vi "Excel Example.vi"() -> ()   [LabVIEW 2017]
doc: "This example shows how to use the LabVIEW NPOI library to manipulate MS Excel Files."
uses:
  LabVIEW NPOI/MS-Excel/MS-Excel.lvclass
  Styles/Underline--ring.ctl
  Styles/Alignment--ring.ctl
  Styles/Font--cluster.ctl
  Styles/Style--cluster.ctl
  LabVIEW NPOI/Document/Read Table As String.vi
  9eaf8ef5-2da6-4511-8777-42b0d28acfa6.vi
  LabVIEW NPOI/Document/Append Table (double).vi
  <vilib>/Utility/sysdir.llb/System Directory Type.ctl
panel:
  in  "print":bool
  in  "HTML File Path":path
  in  "convertToHtml":bool
  out "Read Table Time":u32
  out "Add Table Time":u32
  in  "addImageBttn":bool
  in  "setActiveSheetBttn":bool
  out "Table Control":string[][](table)
  in  "readTableBttn":bool
  in  "Style":u16(ring)
  out "Current Sheet:Next Empty Cell":cluster{"Row":i32, "Column":i32}
  in  "#Columns":i32=100
  in  "#Rows":i32=2
  in  "tableType":enum32{"Strings", "Doubles"}(radio)
  in  "addTableBttn":bool
  in  "Set as active (T)":bool
  in  "addWorksheetBttn":bool
  out "Current Sheet:Name":string
  out "Workbook:Sheet List":string[](array[string])
  out "FilePath":path
  in  "openWorkbookBttn":bool
  in  "baseWorkbookPath":path caption="Folder Path"
  in  "saveAsWorkbookBttn":bool
  in  "saveWorkbookBttn":bool
  in  "removeSheetBttn":bool
  in  "workbookName":string="Book1.xlsx" caption="Name"
  in  "newWorksheetName":string caption="Sheet Name"
  in  "createWorkbookBttn":bool
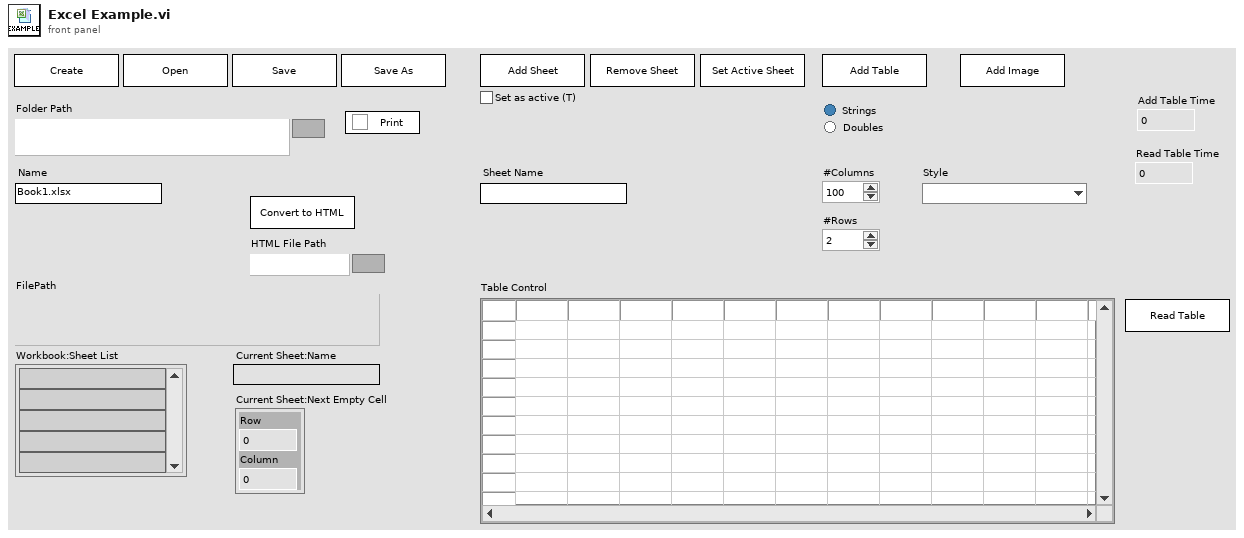
[diagram p1: front panel]
types:
  T1 = typedef "System Directory Type.ctl" = i32
  T2 = cluster{"workbookObject":refnum<class "MS-Excel.lvclass">, "workbookPath":path, "workbookName":string, "worksheetName":string, "styleName":string, "ctlRefs":refnum<vi>[]}
  T3 = typedef "Styles.lvlib/Style--cluster.ctl" = cluster{"Name":string, "Font":T4}
  T4 = typedef "Styles.lvlib/Font--cluster.ctl" = cluster{"Name":string, "Size":i32, "Bold":bool, "Italic":bool, "Underline":T5, "Strike":bool, "Color":u32, "Alignment":T6}
  T5 = typedef "Styles.lvlib/Underline--ring.ctl" = i32
  T6 = typedef "Styles.lvlib/Alignment--ring.ctl" = i32
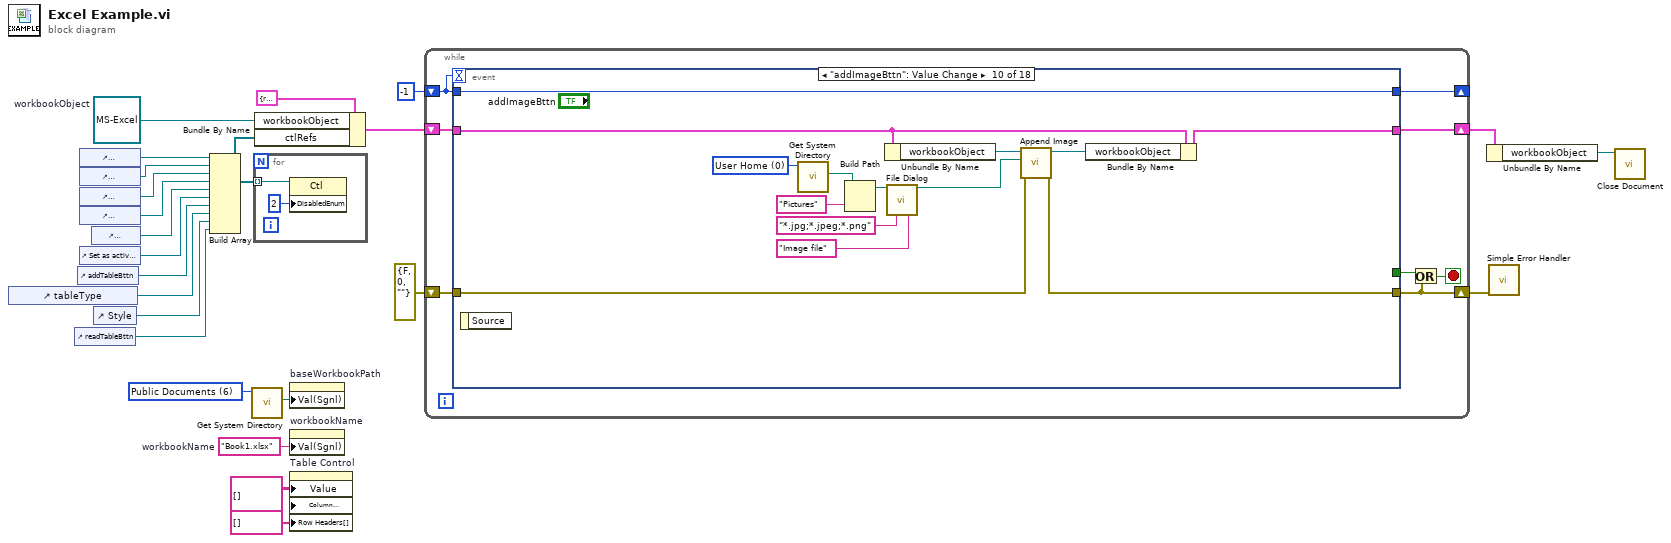
[diagram p0: block diagram]
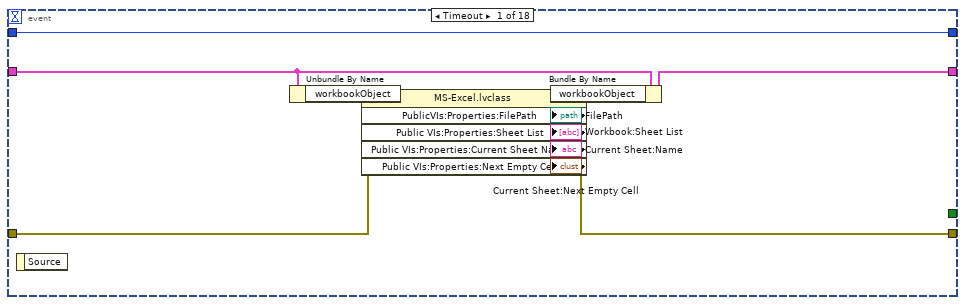
[diagram p2: hidden frame]
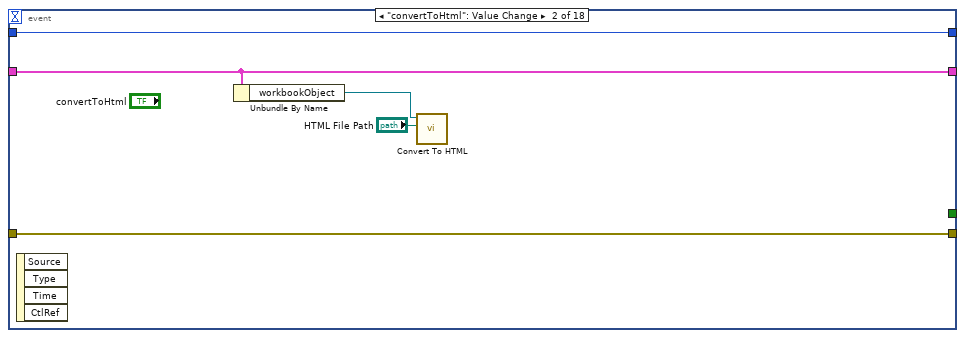
[diagram p3: hidden frame]
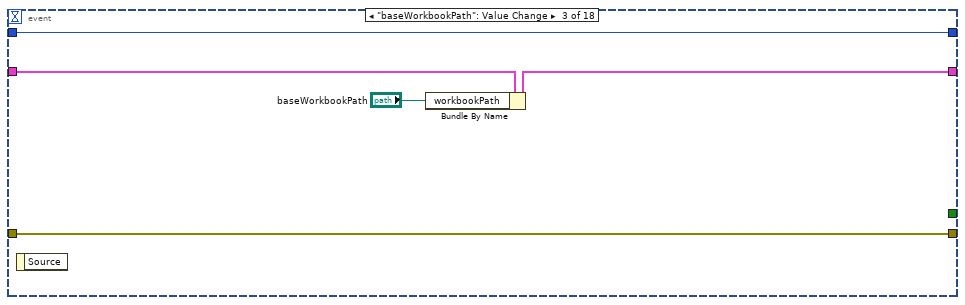
[diagram p4: hidden frame]
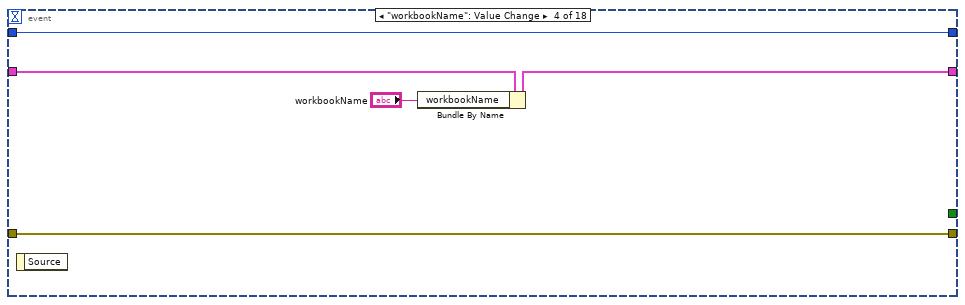
[diagram p5: hidden frame]
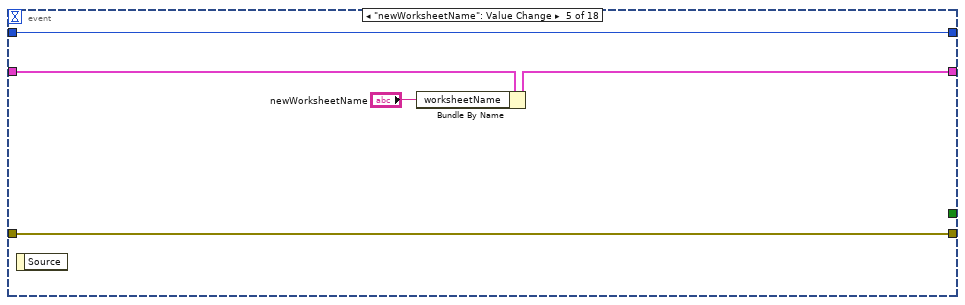
[diagram p6: hidden frame]
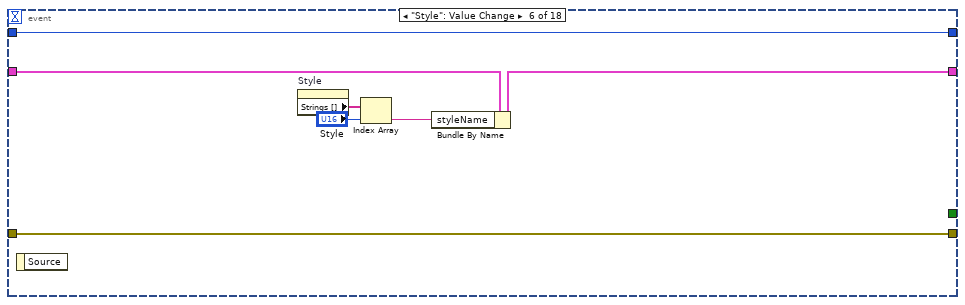
[diagram p7: hidden frame]
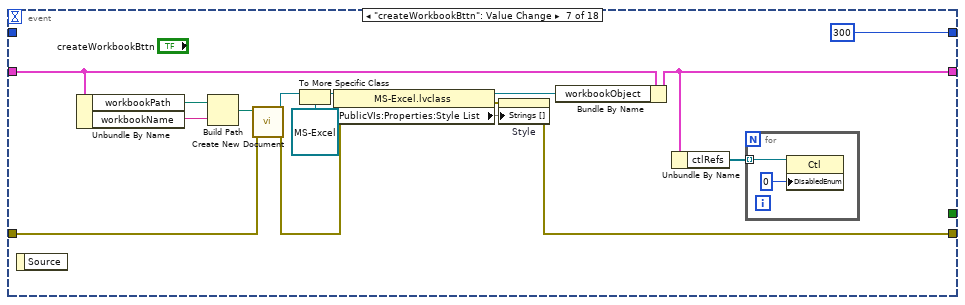
[diagram p8: hidden frame]
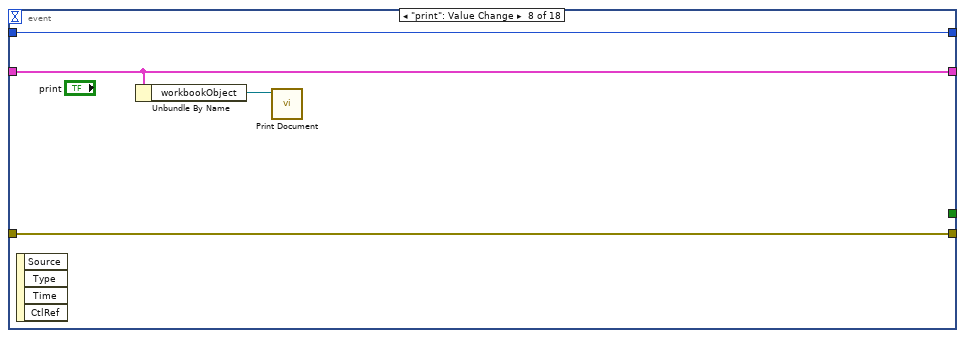
[diagram p9: hidden frame]
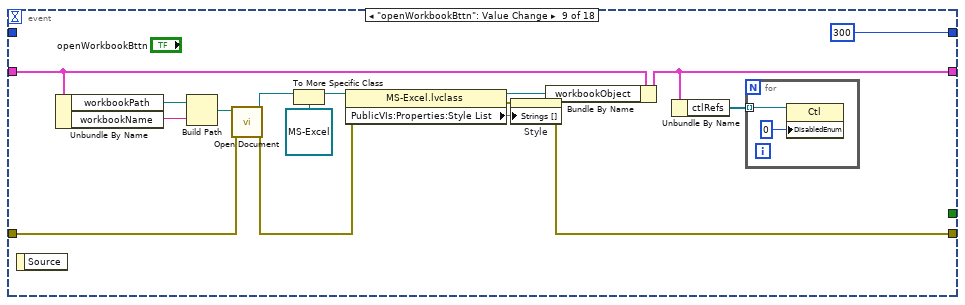
[diagram p10: hidden frame]
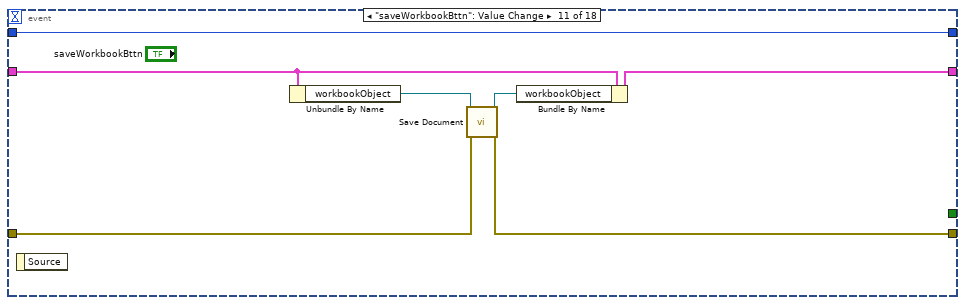
[diagram p11: hidden frame]
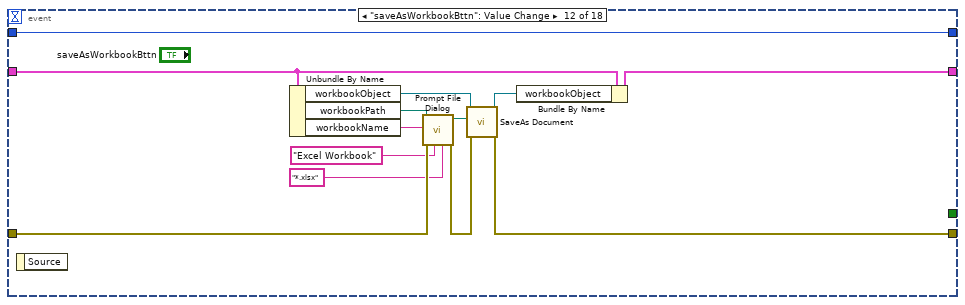
[diagram p12: hidden frame]
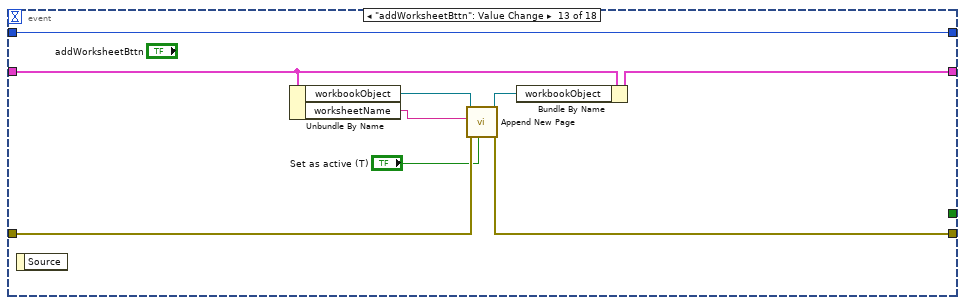
[diagram p13: hidden frame]
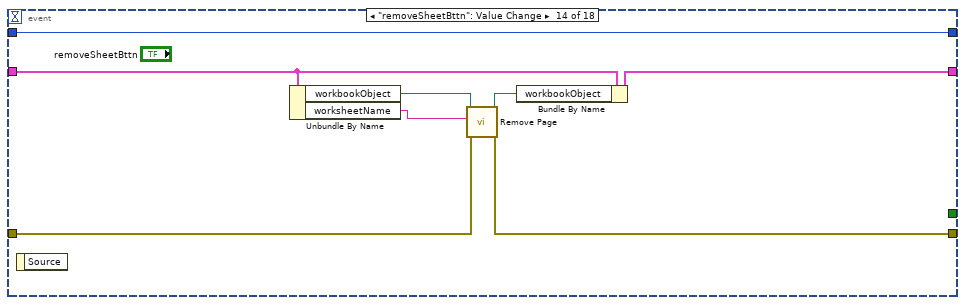
[diagram p14: hidden frame]
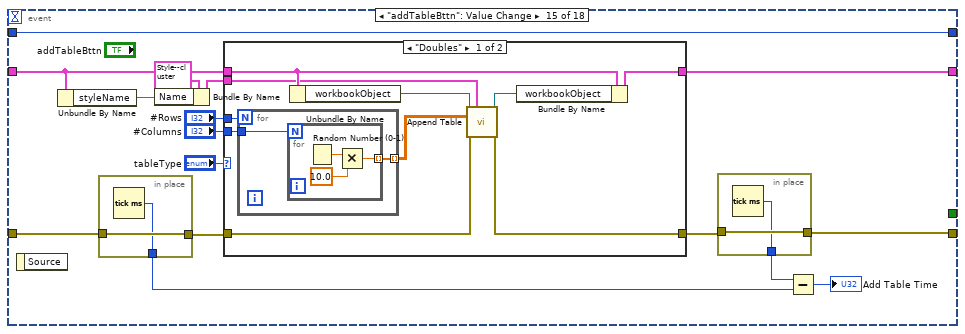
[diagram p15: hidden frame]
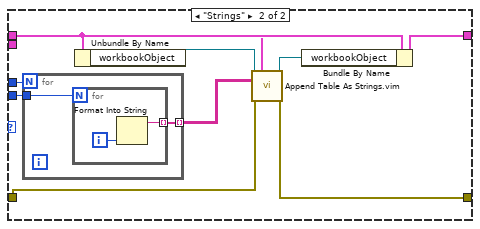
[diagram p16: hidden frame]
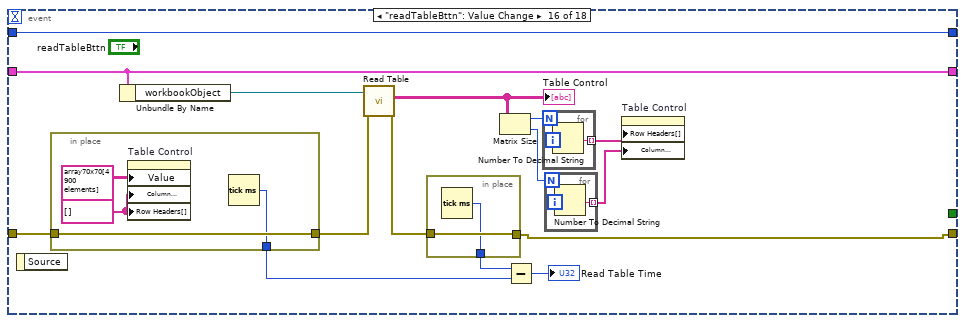
[diagram p17: hidden frame]
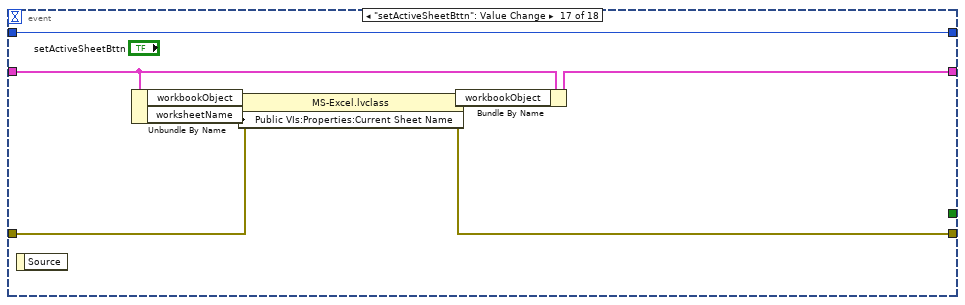
[diagram p18: hidden frame]
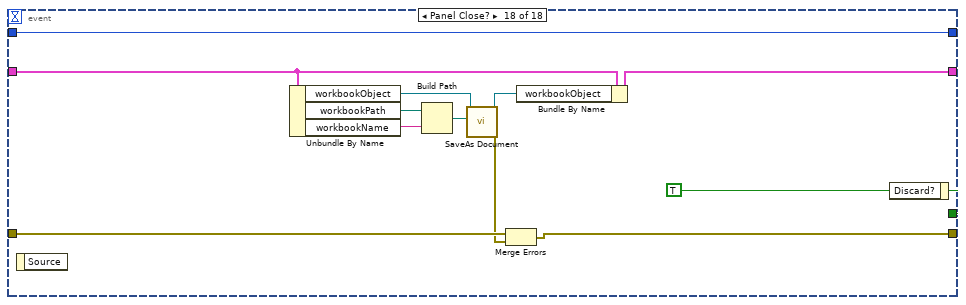
[diagram p19: hidden frame]
diagram:
  w2 = T1 6 items=["User Home"=0, "User Desktop"=1, "User Documents"=2, "User Application Data"=3, "User Preferences"=4, "User Temporary"=5, "Public Documents"=6, "Public Application Data"=7, "Public Preferences"=8, "Public Cache"=13, "System Core Libraries"=9, "System Installed Libraries"=10, "Application Files"=11, "Boot Volume Root"=12] ("system directory type")
  w3 = string[] [] ("Row Header Strings[]")
  w9 = "Book1.xlsx"  # workbookName
  w17 = refnum<class "MS-Excel.lvclass"> refnum  # workbookObject
  n1 = control-ref of="tableType"() -> (w7:refnum<vi>)
  n2 = control-ref of="readTableBttn"() -> (w5:refnum<vi>)
  n3 = control-ref of="addTableBttn"() -> (w8:refnum<vi>)
  n4 = control-ref of="saveWorkbookBttn"() -> (w16:refnum<vi>)
  n5 = control-ref of="saveAsWorkbookBttn"() -> (w15:refnum<vi>)
  n6 = control-ref of="addWorksheetBttn"() -> (w14:refnum<vi>)
  n7 = control-ref of="removeSheetBttn"() -> (w13:refnum<vi>)
  n8 = control-ref of="Set as active (T)"() -> (w11:refnum<vi>)
  n9 = control-ref of="newWorksheetName"() -> (w12:refnum<vi>)
  n10 = control-ref of="Style"() -> (w6:refnum<vi>)
  n11 = Build Array(w16, w15, w14, w13, w12, w11, w8, w7, w6, w5) -> (w10:refnum<vi>[])
  n12 = call <vilib>:"Get System Directory.vi"("system directory type"=w2) -> ("system directory"=w1:path)  [unwired: 10 in]
  n13 = for {
    tunnel: w10 -> [w26] mode=indexing
    n14 = property class="Ctl"(reference=w26, "DisabledEnum"=u8 2) -> ()  [unwired: 1 in, 2 out]
  }
  n15 = Bundle By Name(cluster=T2 {"workbookObject"=refnum, "workbookPath"=path "", "workbookName"="", "worksheetName"="", "styleName"="Default", "ctlRefs"=[]}, "workbookObject"=w17, "ctlRefs"=w10) -> (w24:T2)
  n16 = property on="baseWorkbookPath" class="Path"("Val(Sgnl)"=w1) -> ()  [unwired: 2 in, 2 out]
  n17 = property on="workbookName" class="Str"("Val(Sgnl)"=w9) -> ()  [unwired: 2 in, 2 out]
  n18 = property on="Table Control" class="Tbl (strict)"("Value"=string[][] [] ("Table Control"), "Column Headers[]"=w3, "Row Headers[]"=w3) -> ()  [unwired: 2 in, 2 out]
  n19 = while {
    shift-right: [w33] -> w20
    shift-left: w24 -> [w34]
    shift-right: [w31] -> w23
    shift-left: errorcluster {"status"=FALSE, "code"=0, "source"=""} ("error IO") -> [w32]
    shift-right: [w27] -> _
    shift-left: -1 -> [w28]
    stop <- w29 stop-if-true
    n20 = event shown="[9] \"addImageBttn\": Value Change" {
      selector: _ -> [_ _ _ _ _ _ _ _ _ _ _ _ _ _ _ _ _ _]
      dyn-events: _ -> [_ _ _ _ _ _ _ _ _ _ _ _ _ _ _ _ _ _]
      timeout: w28 -> [_ _ _ _ _ _ _ _ _ _ _ _ _ _ _ _ _ _]
      tunnel: [_ _ _ _ _ _ _ _ _ _ _ _ _ _ _ _ _ w250] -> w30
      tunnel: w34 -> [w45 w48 w55 w60 w65 w72 w88 w92 w110 w125 w133 w146 w155 w163 w174 w226 w244 w257]
      tunnel: [w36 w48 w54 w59 w63 w70 w82 w92 w105 w121 w131 w144 w153 w161 w179 w226 w239 w252] -> w33
      tunnel: [w41 w50 w52 w57 w64 w71 w76 w94 w99 w122 w129 w142 w151 w159 w167 w216 w240 w248] -> w31
      tunnel: w32 -> [w42 w50 w52 w57 w64 w71 w84 w94 w107 w123 w128 w140 w150 w158 w170 w219 w241 w249]
      tunnel: w28 -> [w37 w49 w51 w56 w61 w69 _ w93 _ w126 w127 w134 w148 w156 w178 w227 w245 w246]
      tunnel: [w37 w49 w51 w56 w61 w69 300 w93 300 w126 w127 w134 w148 w156 w178 w227 w245 w246] -> w27
      event Timeout {
        n21 = event-data() -> ()  [unwired: 1 in, 1 out]
        n22 = Unbundle By Name(w45) -> ("workbookObject"=w44:refnum<class "MS-Excel.lvclass">)
        n23 = property class="MS-Excel.lvclass"(reference=w44, error in=w42) -> (reference out=w43:refnum<class "MS-Excel.lvclass">, error out=w41:errorcluster, "PublicVIs:Properties:FilePath"=→"FilePath", "Public VIs:Properties:Sheet List"=→"Workbook:Sheet List", "Public VIs:Properties:Current Sheet Name"=→"Current Sheet:Name", "Public VIs:Properties:Next Empty Cell"=→"Current Sheet:Next Empty Cell")
        n24 = Bundle By Name(cluster=w45, "workbookObject"=w43) -> (w36:T2)
      }
      event "convertToHtml": Value Change {
        n25 = event-data() -> ()  [unwired: 1 in, 4 out]
        n26 = Unbundle By Name(w48) -> ("workbookObject"=w47:refnum<class "MS-Excel.lvclass">)
        n27 = call "Convert To HTML.vi"("HTML File Path"="HTML File Path", "Document in"=w47) -> ()  [unwired: 8 in, 2 out]
      }
      event "baseWorkbookPath": Value Change {
        n28 = event-data() -> ()  [unwired: 1 in, 1 out]
        n29 = Bundle By Name(cluster=w55, "workbookPath"="baseWorkbookPath") -> (w54:T2)
      }
      event "workbookName": Value Change {
        n30 = event-data() -> ()  [unwired: 1 in, 1 out]
        n31 = Bundle By Name(cluster=w60, "workbookName"="workbookName") -> (w59:T2)
      }
      event "newWorksheetName": Value Change {
        n32 = event-data() -> ()  [unwired: 1 in, 1 out]
        n33 = Bundle By Name(cluster=w65, "worksheetName"="newWorksheetName") -> (w63:T2)
      }
      event "Style": Value Change {
        n34 = event-data() -> ()  [unwired: 1 in, 1 out]
        n35 = property on="Style" class="Ring (strict)"() -> ("Strings []"=w68:string[])  [unwired: 2 in, 2 out]
        n36 = Index Array(array=w68, index="Style") -> (element=w67:string)
        n37 = Bundle By Name(cluster=w72, "styleName"=w67) -> (w70:T2)
      }
      event "createWorkbookBttn": Value Change {
        n38 = event-data() -> ()  [unwired: 1 in, 1 out]
        n39 = Unbundle By Name(w88) -> ("workbookPath"=w87:path, "workbookName"=w86:string)
        n40 = Build Path(base path=w87, name or relative path=w86) -> (appended path=w75:path)
        n41 = call "Create New Document.vi"("error in (no error)"=w84, "File Path"=w75) -> ("error out"=w79:errorcluster, "Document out"=w85:refnum<class "Document.lvclass">)  [unwired: 8 in]
        n42 = To More Specific Class(target class=refnum<class "MS-Excel.lvclass"> refnum ("workbookObject"), reference=w85) -> (specific class reference=w74:refnum<class "MS-Excel.lvclass">)  [unwired: 1 in, 1 out]
        n43 = property class="MS-Excel.lvclass"(reference=w74, error in=w79) -> (reference out=w80:refnum<class "MS-Excel.lvclass">, error out=w77:errorcluster, "PublicVIs:Properties:Style List"=w78)
        n44 = property on="Style" class="Ring (strict)"(error in=w77, "Strings []"=w78) -> (error out=w76:errorcluster)  [unwired: 1 in, 1 out]
        n45 = Bundle By Name(cluster=w88, "workbookObject"=w80) -> (w82:T2)
        n46 = Unbundle By Name(w82) -> ("ctlRefs"=w81:refnum<vi>[])
        n47 = for {
          tunnel: w81 -> [w90] mode=indexing
          n48 = property class="Ctl"(reference=w90, "DisabledEnum"=u8 0) -> ()  [unwired: 1 in, 2 out]
        }
      }
      event "print": Value Change {
        n49 = event-data() -> ()  [unwired: 1 in, 4 out]
        n50 = Unbundle By Name(w92) -> ("workbookObject"=w91:refnum<class "MS-Excel.lvclass">)
        n51 = call "Print Document.vi"("Document in"=w91) -> ()  [unwired: 9 in, 2 out]
      }
      event "openWorkbookBttn": Value Change {
        n52 = event-data() -> ()  [unwired: 1 in, 1 out]
        n53 = Unbundle By Name(w110) -> ("workbookPath"=w109:path, "workbookName"=w108:string)
        n54 = Build Path(base path=w109, name or relative path=w108) -> (appended path=w98:path)
        n55 = call "Open Document.vi"("error in (no error)"=w107, "File Path"=w98) -> ("error out"=w101:errorcluster, "Document out"=w96:refnum<class "Document.lvclass">)  [unwired: 8 in]
        n56 = To More Specific Class(target class=refnum<class "MS-Excel.lvclass"> refnum ("workbookObject"), reference=w96) -> (specific class reference=w95:refnum<class "MS-Excel.lvclass">)  [unwired: 1 in, 1 out]
        n57 = property class="MS-Excel.lvclass"(reference=w95, error in=w101) -> (reference out=w102:refnum<class "MS-Excel.lvclass">, error out=w100:errorcluster, "PublicVIs:Properties:Style List"=w103)
        n58 = property on="Style" class="Ring (strict)"(error in=w100, "Strings []"=w103) -> (error out=w99:errorcluster)  [unwired: 1 in, 1 out]
        n59 = Bundle By Name(cluster=w110, "workbookObject"=w102) -> (w105:T2)
        n60 = Unbundle By Name(w105) -> ("ctlRefs"=w104:refnum<vi>[])
        n61 = for {
          tunnel: w104 -> [w112] mode=indexing
          n62 = property class="Ctl"(reference=w112, "DisabledEnum"=u8 0) -> ()  [unwired: 1 in, 2 out]
        }
      }
      event "addImageBttn": Value Change {
        w115 = T1 0 items=["User Home"=0, "User Desktop"=1, "User Documents"=2, "User Application Data"=3, "User Preferences"=4, "User Temporary"=5, "Public Documents"=6, "Public Application Data"=7, "Public Preferences"=8, "Public Cache"=13, "System Core Libraries"=9, "System Installed Libraries"=10, "Application Files"=11, "Boot Volume Root"=12] ("system directory type")
        n63 = event-data() -> ()  [unwired: 1 in, 1 out]
        n64 = call <vilib>:"Get System Directory.vi"("system directory type"=w115) -> ("system directory"=w116:path)  [unwired: 10 in]
        n65 = Build Path(base path=w116, name or relative path="Pictures") -> (appended path=w114:path)
        n66 = Unbundle By Name(w125) -> ("workbookObject"=w124:refnum<class "MS-Excel.lvclass">)
        n67 = call "File Dialog"("start path"=w114, "pattern (all files)"="*.jpg;*.jpeg;*.png", "pattern label"="Image file") -> ("selected path"=w119:path)  [unwired: 9 in, 3 out]
        n68 = call "Append Image.vi"("error in (no error)"=w123, "Image File Path"=w119, "Document in"=w124) -> ("error out"=w122:errorcluster, "Document out"=w120:refnum<class "MS-Excel.lvclass">)  [unwired: 7 in]
        n69 = Bundle By Name(cluster=w125, "workbookObject"=w120) -> (w121:T2)
      }
      event "saveWorkbookBttn": Value Change {
        n70 = event-data() -> ()  [unwired: 1 in, 1 out]
        n71 = Unbundle By Name(w133) -> ("workbookObject"=w132:refnum<class "MS-Excel.lvclass">)
        n72 = call "Save Document.vi"("error in (no error)"=w128, "Document in"=w132) -> ("error out"=w129:errorcluster, "Document out"=w130:refnum<class "MS-Excel.lvclass">)  [unwired: 8 in]
        n73 = Bundle By Name(cluster=w133, "workbookObject"=w130) -> (w131:T2)
      }
      event "saveAsWorkbookBttn": Value Change {
        n74 = event-data() -> ()  [unwired: 1 in, 1 out]
        n75 = Unbundle By Name(w146) -> ("workbookObject"=w145:refnum<class "MS-Excel.lvclass">, "workbookPath"=w136:path, "workbookName"=w135:string)
        n76 = call "Prompt File Dialog.vi"("pattern (all files)"="*.xlsx", "pattern label"="Excel Workbook", "error in"=w140, "default name"=w135, "File Path"=w136) -> ("error out"=w139:errorcluster, "selected path"=w141:path)  [unwired: 5 in]
        n77 = call "SaveAs Document.vi"("error in (no error)"=w139, "File Path"=w141, "Document in"=w145) -> ("error out"=w142:errorcluster, "Document out"=w143:refnum<class "MS-Excel.lvclass">)  [unwired: 7 in]
        n78 = Bundle By Name(cluster=w146, "workbookObject"=w143) -> (w144:T2)
      }
      event "addWorksheetBttn": Value Change {
        n79 = event-data() -> ()  [unwired: 1 in, 1 out]
        n80 = Unbundle By Name(w155) -> ("workbookObject"=w154:refnum<class "MS-Excel.lvclass">, "worksheetName"=w149:string)
        n81 = call "Append New Page.vi"("Set as active (T)"="Set as active (T)", "error in (no error)"=w150, "Page Name"=w149, "Document in"=w154) -> ("error out"=w151:errorcluster, "Document out"=w152:refnum<class "MS-Excel.lvclass">)  [unwired: 4 in, 2 out]
        n82 = Bundle By Name(cluster=w155, "workbookObject"=w152) -> (w153:T2)
      }
      event "removeSheetBttn": Value Change {
        n83 = event-data() -> ()  [unwired: 1 in, 1 out]
        n84 = Unbundle By Name(w163) -> ("workbookObject"=w162:refnum<class "MS-Excel.lvclass">, "worksheetName"=w157:string)
        n85 = call "Remove Page.vi"("error in (no error)"=w158, "Page Name"=w157, "Document in"=w162) -> ("error out"=w159:errorcluster, "Document out"=w160:refnum<class "MS-Excel.lvclass">)  [unwired: 7 in]
        n86 = Bundle By Name(cluster=w163, "workbookObject"=w160) -> (w161:T2)
      }
      event "addTableBttn": Value Change {
        n87 = event-data() -> ()  [unwired: 1 in, 1 out]
        n88 = Unbundle By Name(w174) -> ("styleName"=w171:string)
        n89 = in-place {
          in-place-border: w170 -> [w183]
          in-place-border: [w183] -> w169
          in-place-border: [w182] -> w165
          n90 = Tick Count (ms)() -> (millisecond timer value=w182:u32)
        }
        n91 = Bundle By Name(cluster=T3 {"Name"="Default", "Font"={"Name"="Calibri", "Size"=12, "Bold"=FALSE, "Italic"=FALSE, "Underline"=18, "Strike"=FALSE, "Color"=0, "Alignment"=1}} ("Style"), "Name"=w171) -> (w172:T3)
        n92 = case shown="\"Doubles\"" "tableType" {
          tunnel: w174 -> [w193 w208]
          tunnel: [w191 w206] -> w179
          tunnel: [w189 w204] -> w168
          tunnel: w169 -> [w188 w203]
          tunnel: "#Columns" -> [w185 w201]
          tunnel: "#Rows" -> [w186 w200]
          tunnel: w172 -> [w184 w199]
          frame "Doubles" {
            n93 = for {
              N: w186 -> [_]
              tunnel: [w195] -> w187 mode=indexing
              tunnel: w185 -> [w194]
              n94 = for {
                N: w194 -> [_]
                tunnel: [w197] -> w195 mode=indexing
                n95 = Random Number (0-1)() -> (number: 0 to 1=w198:dbl)
                n96 = Multiply(x=w198, y=10.0) -> (x*y=w197:dbl)
              }
            }
            n97 = Unbundle By Name(w193) -> ("workbookObject"=w192:refnum<class "MS-Excel.lvclass">)
            n98 = call-poly "Append Table.vi"("Document in"=w192, "Style"=w184, "Table"=w187, "error in (no error)"=w188) -> ("Document out"=w190:refnum<class "MS-Excel.lvclass">, "error out"=w189:errorcluster)  [unwired: 10 in]
            n99 = Bundle By Name(cluster=w193, "workbookObject"=w190) -> (w191:T2)
          }
          frame "Strings" {
            n100 = for {
              N: w200 -> [_]
              tunnel: [w210] -> w202 mode=indexing
              tunnel: w201 -> [w209]
              n101 = for {
                N: w209 -> [_]
                tunnel: [w211] -> w210 mode=indexing
                i -> [w212]
                n102 = Format Into String(w212) -> (resulting string=w211:string)  [unwired: 3 in, 1 out]
              }
            }
            n103 = Unbundle By Name(w208) -> ("workbookObject"=w207:refnum<class "MS-Excel.lvclass">)
            n104 = call "Append Table As Strings.vim"("Document in"=w207, "Style"=w199, "Table"=w202, "error in (no error)"=w203) -> ("Document out"=w205:refnum<class "MS-Excel.lvclass">, "error out"=w204:errorcluster)  [unwired: 10 in]
            n105 = Bundle By Name(cluster=w208, "workbookObject"=w205) -> (w206:T2)
          }
        }
        n106 = in-place {
          in-place-border: w168 -> [w181]
          in-place-border: [w181] -> w167
          in-place-border: [w180] -> w166
          n107 = Tick Count (ms)() -> (millisecond timer value=w180:u32)
        }
        n108 = Subtract(x=w166, y=w165) -> (x-y=→"Add Table Time":u32)
      }
      event "readTableBttn": Value Change {
        n109 = event-data() -> ()  [unwired: 1 in, 1 out]
        n110 = in-place {
          in-place-border: w219 -> [w231]
          in-place-border: [w231] -> w218
          in-place-border: [w230] -> w214
          w233 = string[] [] ("Row Header Strings[]")
          n111 = property on="Table Control" class="Tbl (strict)"("Value"=string[][] array70x70[4900 elements] ("Table Control"), "Column Headers[]"=w233, "Row Headers[]"=w233) -> ()  [unwired: 2 in, 2 out]
          n112 = Tick Count (ms)() -> (millisecond timer value=w230:u32)
        }
        n113 = Unbundle By Name(w226) -> ("workbookObject"=w225:refnum<class "MS-Excel.lvclass">)
        n114 = call-poly "Read Table.vi"("error in (no error)"=w218, "Document in"=w225) -> ("error out"=w217:errorcluster, "Table As String"=w224:string[][])  [unwired: 7 in, 1 out]
        "Table Control" <- w224
        n115 = in-place {
          in-place-border: w217 -> [w229]
          in-place-border: [w229] -> w216
          in-place-border: [w228] -> w215
          n116 = Tick Count (ms)() -> (millisecond timer value=w228:u32)
        }
        n117 = Matrix Size(0:w224) -> (1:w223:i32, 2:w221:i32)
        n118 = Subtract(x=w215, y=w214) -> (x-y=→"Read Table Time":u32)
        n119 = for {
          N: w223 -> [_]
          tunnel: [w236] -> w222 mode=indexing
          i -> [w237]
          n120 = Number To Decimal String(number=w237) -> (decimal integer string=w236:string)  [unwired: 1 in]
        }
        n121 = for {
          N: w221 -> [_]
          tunnel: [w234] -> w220 mode=indexing
          i -> [w235]
          n122 = Number To Decimal String(number=w235) -> (decimal integer string=w234:string)  [unwired: 1 in]
        }
        n123 = property on="Table Control" class="Tbl (strict)"("Row Headers[]"=w222, "Column Headers[]"=w220) -> ()  [unwired: 2 in, 2 out]
      }
      event "setActiveSheetBttn": Value Change {
        n124 = event-data() -> ()  [unwired: 1 in, 1 out]
        n125 = Unbundle By Name(w244) -> ("workbookObject"=w243:refnum<class "MS-Excel.lvclass">, "worksheetName"=w242:string)
        n126 = property class="MS-Excel.lvclass"(reference=w243, error in=w241, "Public VIs:Properties:Current Sheet Name"=w242) -> (reference out=w238:refnum<class "MS-Excel.lvclass">, error out=w240:errorcluster)
        n127 = Bundle By Name(cluster=w244, "workbookObject"=w238) -> (w239:T2)
      }
      event Panel Close? {
        w250 = TRUE ("Discard?")
        n128 = event-data() -> ()  [unwired: 1 in, 1 out]
        n129 = Unbundle By Name(w257) -> ("workbookObject"=w254:refnum<class "MS-Excel.lvclass">, "workbookPath"=w256:path, "workbookName"=w255:string)
        n130 = Build Path(base path=w256, name or relative path=w255) -> (appended path=w253:path)
        n131 = call "SaveAs Document.vi"("File Path"=w253, "Document in"=w254) -> ("error out"=w247:errorcluster, "Document out"=w251:refnum<class "MS-Excel.lvclass">)  [unwired: 8 in]
        n132 = Merge Errors(w249, w247) -> (w248:errorcluster)
        n133 = Bundle By Name(cluster=w257, "workbookObject"=w251) -> (w252:T2)
        n134 = event-data("Discard?"=w250) -> ()  [unwired: 1 in, 1 out]
      }
    }
    n135 = Or(x=w30, y=w31) -> (x .or. y?=w29:bool)
  }
  n136 = Unbundle By Name(w20) -> ("workbookObject"=w19:refnum<class "MS-Excel.lvclass">)
  n137 = call <vilib>:"Simple Error Handler.vi"("error in (no error)"=w23) -> ()  [unwired: 4 in, 5 out]
  n138 = call "Close Document.vi"("Document in"=w19) -> ()  [unwired: 10 in, 1 out]
